vi "Read-Async-with-TypeResolving-Sensata.vi"() -> ()   [LabVIEW 2020]
doc: "ADS Asynchronous read example using preconfigured blocks. \n\nThe client reads data asynchronously and does not wait for the respose from server."
uses:
  <userlib>/Beckhoff-LabVIEW-Interface/_DependsOn/TypeDefs/Low-Levels/Symbol Interface Mode.ctl
  <userlib>/Beckhoff-LabVIEW-Interface/_DependsOn/Base/Read/Read Async.vi
  <userlib>/Beckhoff-LabVIEW-Interface/_DependsOn/Base/TypeResolver/Get TypeResolver.vi
panel:
  out "Iterations":i32
  out "Data":variant
  in  "Symbol file path":path
  out "Read Status?":bool
  # "The example starts with retrieving read\nADS Symbols and selects the first symbol. The symbol can be selected:\n- Using Symbol file in symbol file path\n- Using Symbol Interface (UI), which is opened automatically if file path is empty.\n\nThe example reads the selected symbol, only once, asynchronously and does not wait for ADS response. Iterations demonstrates how many calls it takes to successfully read the data package. \n\nThe example uses TypeResolver to convert ADS row data to LabVIEW™ type.\n\nFor more information, please refer to block diagram comments."
  # "Note: This example is only an illustration of all possible ways\nhow this Product can be used."
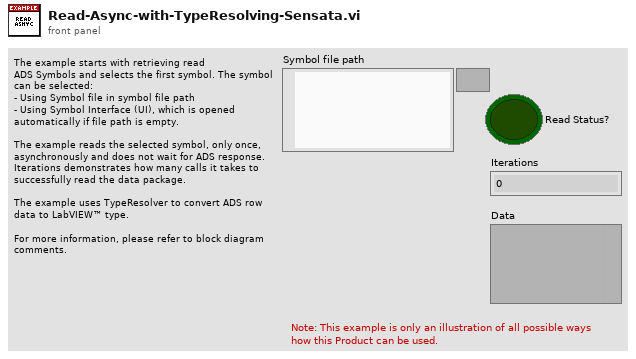
[diagram p1: front panel]
types:
  T1 = typedef "Symbol Interface Mode.ctl" = enum16{"Read Only", "Write Only", "Read & Write"}
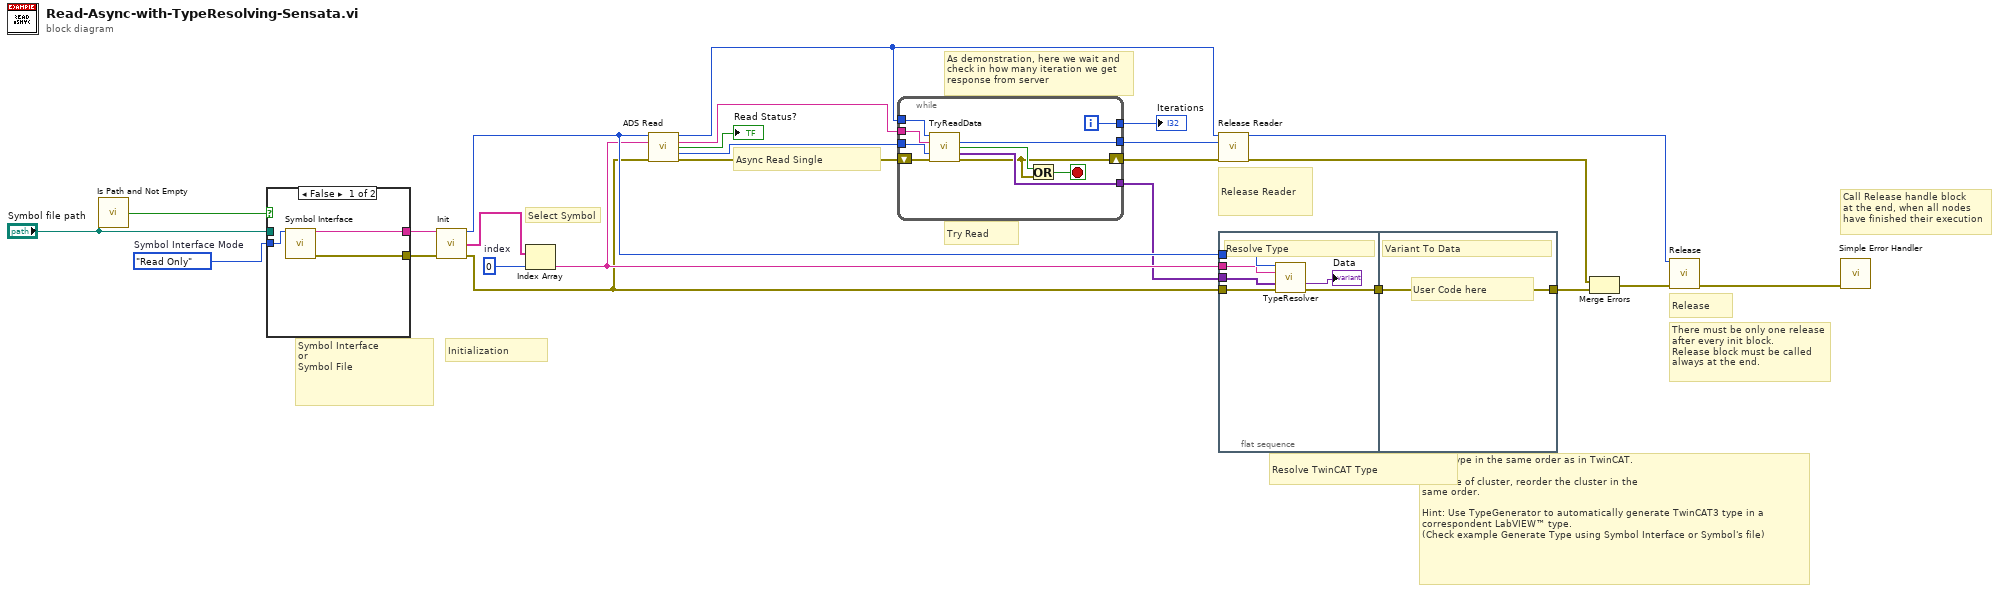
[diagram p0: block diagram]
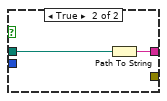
[diagram p2: hidden frame]
diagram:
  w2 = Symbol_Interface_Mode."Read Only"  # Symbol Interface Mode
  w25 = 0  # index
  # "Build Type in the same order as in TwinCAT.\n\n- In case of cluster, reorder the cluster in the\nsame order.\n\nHint: Use TypeGenerator to automatically generate TwinCAT3 type in a correspondent LabVIEW™ type.\n(Check example Generate Type using Symbol Interface or Symbol's file)"
  # "Symbol Interface\nor\nSymbol File"
  # "Release Reader"
  # "As demonstration, here we wait and \ncheck in how many iteration we get\nresponse from server"
  # "Call Release handle block\nat the end, when all nodes\nhave finished their execution"
  # "There must be only one release\nafter every init block.\nRelease block must be called\nalways at the end."
  # "Try Read"
  # "Select Symbol"
  # "Async Read Single"
  # "Resolve TwinCAT Type"
  # "Release"
  # "Initialization"
  n1 = call <vilib>:"Is Path and Not Empty.vi"("path"="Symbol file path") -> ("Is Path and Not Empty?"=w6:bool)  [unwired: 4 in]
  n2 = case shown="False" w6 {
    tunnel: [w28 w30] -> w4
    tunnel: "Symbol file path" -> [_ w29]
    tunnel: [w27 _] -> w3
    tunnel: w2 -> [w26 _]
    frame False {
      n3 = call <userlib>:"Symbol Interface.vi"("Symbol Interface Mode"=w26) -> ("PortInfo"=w28:string, "error out"=w27:errorcluster)  [unwired: 13 in]
    }
    frame True {
      n4 = Path To String(path=w29) -> (string=w30:string)
    }
  }
  n5 = call <userlib>:"Init.vi"("XMLDescription"=w4, "error in (no error)"=w3) -> ("Handle"=w20:u32, "ReadGrpSymbols"=w23:string[], "error out"=w18:errorcluster)  [unwired: 9 in, 2 out]
  n6 = Index Array "Index Array"(array=w23, index=w25) -> (element=w19:string)
  n7 = call-poly <userlib>:"ADS Read.vi"("Handle"=w20, "SymbolName"=w19, "error in (no error)"=w18) -> ("Handle"=w9:u32, "SymbolName"=w12:string, "Read Status"=→"Read Status?":bool, "ReadHdl"=w17:u32, "error out"=w16:errorcluster)  [unwired: 8 in]
  n8 = while {
    tunnel: w17 -> [w39]
    shift-right: [w34] -> w11
    shift-left: w16 -> [w37]
    tunnel: [w38] -> w14
    tunnel: [w40] -> w15
    tunnel: w9 -> [w33]
    tunnel: w12 -> [w32]
    tunnel: [w31] -> w8
    i -> [w40]
    stop <- w36 stop-if-true
    n9 = call <userlib>:"TryReadData.vi"("Handle"=w33, "SymbolName"=w32, "ReadHandle"=w39, "error in"=w37) -> ("ReadHandle"=w31:u32, "Read status?"=w35:bool, "Ads Read Data"=w38:variant[], "error out"=w34:errorcluster)  [unwired: 7 in, 1 out]
    n10 = Or(x=w35, y=w34) -> (x .or. y?=w36:bool)
  }
  "Iterations" <- w15
  n11 = call <userlib>:"Release Reader.vi"("Handle"=w9, "ReadHandle"=w8, "error in (no error)"=w11) -> ("Handle"=w7:u32, "error out"=w10:errorcluster)  [unwired: 11 in]
  n12 = flat-sequence {
    tunnel: w20 -> [w44]
    tunnel: w19 -> [w43]
    tunnel: w18 -> [w45]
    tunnel: w14 -> [w42]
    tunnel: [w46] -> w13
    tunnel: [w47] -> w24
    tunnel: w13 -> [w47]
    frame #0 {
      # "Resolve Type"
      n13 = call-poly <userlib>:"TypeResolver.vi"("Handle"=w44, "SymbolName"=w43, "ADSRData"=w42, "error in"=w45) -> ("RData"=→"Data":variant, "error out"=w46:errorcluster)  [unwired: 8 in, 2 out]
    }
    frame #1 {
      # "User Code here"
      # "Variant To Data"
    }
  }
  n14 = Merge Errors "Merge Errors"(w10, w24) -> (w21:errorcluster)
  n15 = call <userlib>:"Release.vi"("Handle"=w7, "error in (no error)"=w21) -> ("error out"=w1:errorcluster)  [unwired: 13 in]
  n16 = call <vilib>:"Simple Error Handler.vi"("error in (no error)"=w1) -> ()  [unwired: 4 in, 5 out]
